vi "new_plot.vi"(10 "簇":T1, 11 "配置输入":T2 {"串口通信UI"."Format" items=["标准帧", "扩展帧"]; "串口通信UI"."Type" items=["数据帧", "远程帧"]; "串口通信UI"."ID" format="0x%x"; "串口通信UI"."Fliter" items=["接收所有类型"=1, "只接收标准帧"=2, "只接收扩展帧"=3]; "串口通信UI"."kBaudRate" items=["5k bps"=1, "10k bps"=2, "20k bps"=3, "40k bps"=4, "50k bps"=5, "80k bps"=6, "100k bps"=7, "125k bps"=8, "200k bps"=9, "250k bps"=10, "400k bps"=11, "500k bps"=12, "666k bps"=13, "800k bps"=14, "1000k bps"=15, "33.33k bps"=16, "66.66k bps"=17, "83.33k bps"=18]; "串口通信UI"."Mode" items=["正常工作", "仅侦听模式", "自测模式（环回）"]; "串口通信UI"."InitFlag" items=["使用界面设置参数"=1]; "串口通信UI"."AccMask" format="%08x"; "串口通信UI"."AccCode" format="%08x"; "串口通信UI"."Channel" items=["通道1", "通道2"]; "串口通信UI"."DevType" items=["USB-CAN"=3, "USB-CAN2"=4]; "安全报警UI"."操作 8" items=["产生报警信息（不发声），等待手动操作", "产生报警信息（发声），等待手动操作", "产生报警信息（不发声），自动刹车", "产生报警信息（发声），自动刹车", "产生报警信息（不发声），立即自动断电，开启泄放电阻", "产生报警信息（发声），立即自动断电，开启泄放电阻"]; "安全报警UI"."操作 7" items=["产生报警信息（不发声），等待手动操作", "产生报警信息（发声），等待手动操作", "产生报警信息（不发声），自动刹车", "产生报警信息（发声），自动刹车", "产生报警信息（不发声），立即自动断电，开启泄放电阻", "产生报警信息（发声），立即自动断电，开启泄放电阻"]; "安全报警UI"."操作 6" items=["产生报警信息（不发声），等待手动操作", "产生报警信息（发声），等待手动操作", "产生报警信息（不发声），自动刹车", "产生报警信息（发声），自动刹车", "产生报警信息（不发声），立即自动断电，开启泄放电阻", "产生报警信息（发声），立即自动断电，开启泄放电阻"]; "安全报警UI"."操作 5" items=["产生报警信息（不发声），等待手动操作", "产生报警信息（发声），等待手动操作", "产生报警信息（不发声），自动刹车", "产生报警信息（发声），自动刹车", "产生报警信息（不发声），立即自动断电，开启泄放电阻", "产生报警信息（发声），立即自动断电，开启泄放电阻"]; "安全报警UI"."操作 4" items=["产生报警信息（不发声），等待手动操作", "产生报警信息（发声），等待手动操作", "产生报警信息（不发声），自动刹车", "产生报警信息（发声），自动刹车", "产生报警信息（不发声），立即自动断电，开启泄放电阻", "产生报警信息（发声），立即自动断电，开启泄放电阻"]; "安全报警UI"."操作 3" items=["产生报警信息（不发声），等待手动操作", "产生报警信息（发声），等待手动操作", "产生报警信息（不发声），自动刹车", "产生报警信息（发声），自动刹车", "产生报警信息（不发声），立即自动断电，开启泄放电阻", "产生报警信息（发声），立即自动断电，开启泄放电阻"]; "安全报警UI"."操作 2" items=["产生报警信息（不发声），等待手动操作", "产生报警信息（发声），等待手动操作", "产生报警信息（不发声），自动刹车", "产生报警信息（发声），自动刹车", "产生报警信息（不发声），立即自动断电，开启泄放电阻", "产生报警信息（发声），立即自动断电，开启泄放电阻"]; "安全报警UI"."操作" items=["产生报警信息（不发声），等待手动操作", "产生报警信息（发声），等待手动操作", "产生报警信息（不发声），自动刹车", "产生报警信息（发声），自动刹车", "产生报警信息（不发声），立即自动断电，开启泄放电阻", "产生报警信息（发声），立即自动断电，开启泄放电阻"]}) -> (3 "配置输出":T2 {"串口通信UI"."Format" items=["标准帧", "扩展帧"]; "串口通信UI"."Type" items=["数据帧", "远程帧"]; "串口通信UI"."ID" format="0x%x"; "串口通信UI"."Fliter" items=["接收所有类型"=1, "只接收标准帧"=2, "只接收扩展帧"=3]; "串口通信UI"."kBaudRate" items=["5k bps"=1, "10k bps"=2, "20k bps"=3, "40k bps"=4, "50k bps"=5, "80k bps"=6, "100k bps"=7, "125k bps"=8, "200k bps"=9, "250k bps"=10, "400k bps"=11, "500k bps"=12, "666k bps"=13, "800k bps"=14, "1000k bps"=15, "33.33k bps"=16, "66.66k bps"=17, "83.33k bps"=18]; "串口通信UI"."Mode" items=["正常工作", "仅侦听模式", "自测模式（环回）"]; "串口通信UI"."InitFlag" items=["使用界面设置参数"=1]; "串口通信UI"."AccMask" format="%08x"; "串口通信UI"."AccCode" format="%08x"; "串口通信UI"."Channel" items=["通道1", "通道2"]; "串口通信UI"."DevType" items=["USB-CAN"=3, "USB-CAN2"=4]; "安全报警UI"."操作 8" items=["产生报警信息（不发声），等待手动操作", "产生报警信息（发声），等待手动操作", "产生报警信息（不发声），自动刹车", "产生报警信息（发声），自动刹车", "产生报警信息（不发声），立即自动断电，开启泄放电阻", "产生报警信息（发声），立即自动断电，开启泄放电阻"]; "安全报警UI"."操作 7" items=["产生报警信息（不发声），等待手动操作", "产生报警信息（发声），等待手动操作", "产生报警信息（不发声），自动刹车", "产生报警信息（发声），自动刹车", "产生报警信息（不发声），立即自动断电，开启泄放电阻", "产生报警信息（发声），立即自动断电，开启泄放电阻"]; "安全报警UI"."操作 6" items=["产生报警信息（不发声），等待手动操作", "产生报警信息（发声），等待手动操作", "产生报警信息（不发声），自动刹车", "产生报警信息（发声），自动刹车", "产生报警信息（不发声），立即自动断电，开启泄放电阻", "产生报警信息（发声），立即自动断电，开启泄放电阻"]; "安全报警UI"."操作 5" items=["产生报警信息（不发声），等待手动操作", "产生报警信息（发声），等待手动操作", "产生报警信息（不发声），自动刹车", "产生报警信息（发声），自动刹车", "产生报警信息（不发声），立即自动断电，开启泄放电阻", "产生报警信息（发声），立即自动断电，开启泄放电阻"]; "安全报警UI"."操作 4" items=["产生报警信息（不发声），等待手动操作", "产生报警信息（发声），等待手动操作", "产生报警信息（不发声），自动刹车", "产生报警信息（发声），自动刹车", "产生报警信息（不发声），立即自动断电，开启泄放电阻", "产生报警信息（发声），立即自动断电，开启泄放电阻"]; "安全报警UI"."操作 3" items=["产生报警信息（不发声），等待手动操作", "产生报警信息（发声），等待手动操作", "产生报警信息（不发声），自动刹车", "产生报警信息（发声），自动刹车", "产生报警信息（不发声），立即自动断电，开启泄放电阻", "产生报警信息（发声），立即自动断电，开启泄放电阻"]; "安全报警UI"."操作 2" items=["产生报警信息（不发声），等待手动操作", "产生报警信息（发声），等待手动操作", "产生报警信息（不发声），自动刹车", "产生报警信息（发声），自动刹车", "产生报警信息（不发声），立即自动断电，开启泄放电阻", "产生报警信息（发声），立即自动断电，开启泄放电阻"]; "安全报警UI"."操作" items=["产生报警信息（不发声），等待手动操作", "产生报警信息（发声），等待手动操作", "产生报警信息（不发声），自动刹车", "产生报警信息（发声），自动刹车", "产生报警信息（不发声），立即自动断电，开启泄放电阻", "产生报警信息（发声），立即自动断电，开启泄放电阻"]})   [LabVIEW 2018, in "UI.lvlib"]
uses:
  UI.lvlib
  Settings/Settings.ctl
  Acquisition/Hardware Configuration.ctl
  Acquisition/Signal Type.ctl
  Logging/Logging Configuration.ctl
  Logging/Logging.lvlib
  Acquisition/Acquisition.lvlib
  Settings/Settings.lvlib
panel:
  # "参数配置文件"
  # "输入数据文件"
  # "加载电机"
  # "负载电机"
  # "注：每次运行实验时销毁现有所有图像"
  # "参数配置文件"
  # "输入数据文件"
  # "加载电机"
  # "负载电机"
  # "注：每次运行实验时销毁现有所有图像"
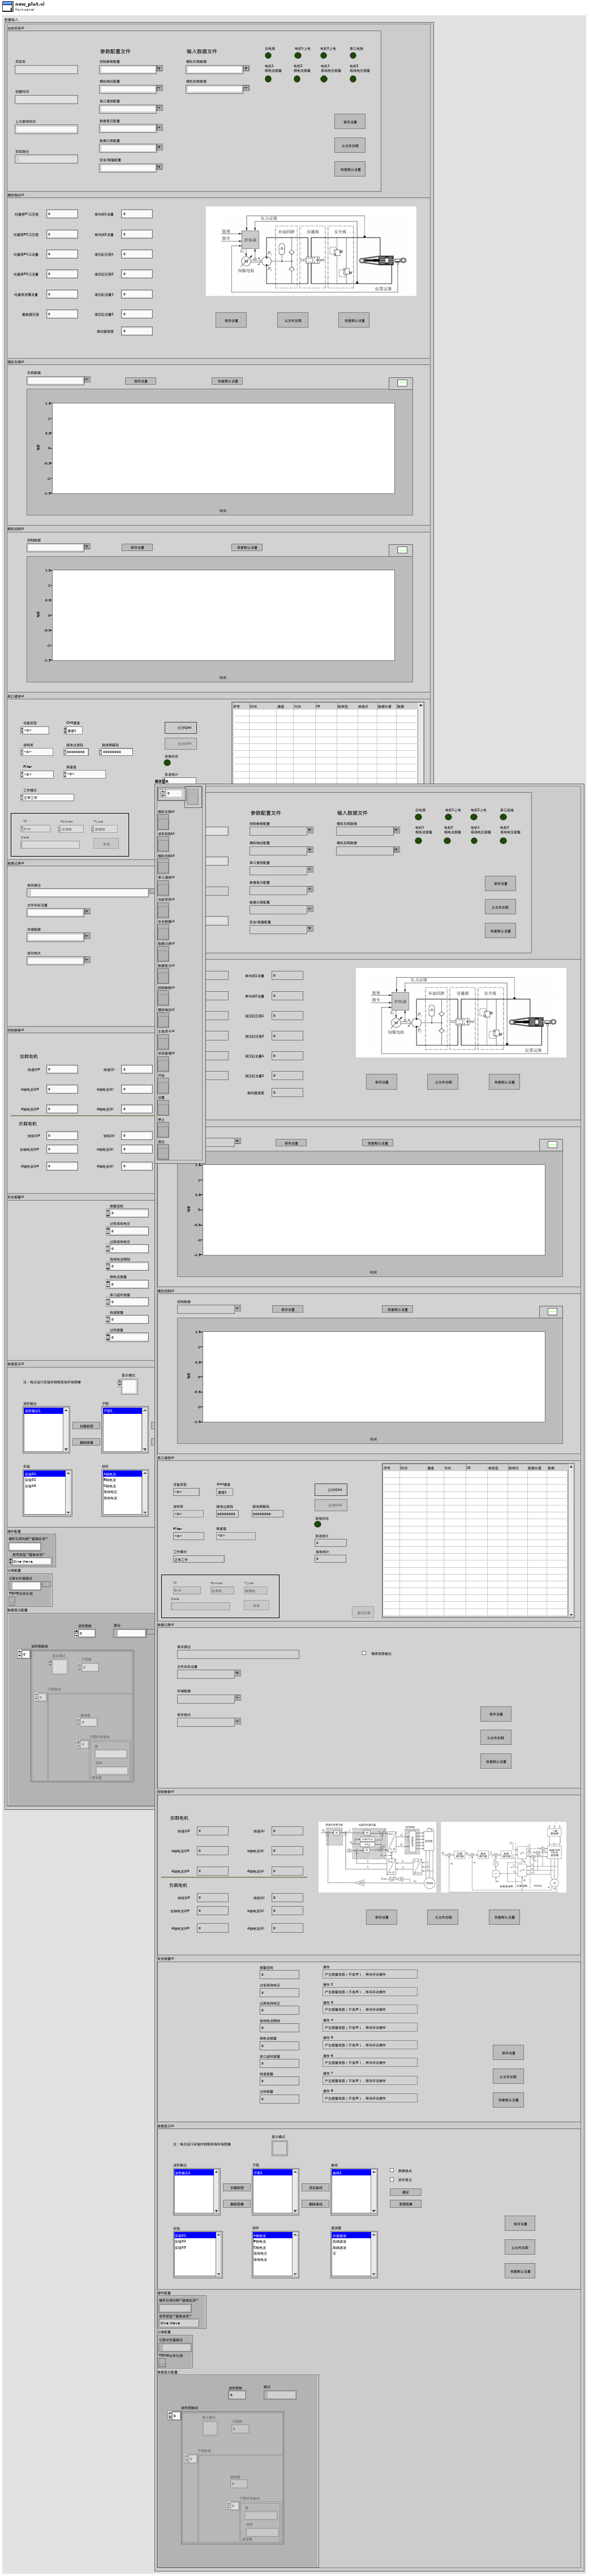
[diagram p1: front panel]
types:
  T1 = typedef "引用簇.ctl" = cluster{"数组":refnum<vi>[], "模拟负载UI":refnum<vi>, "波形控制UI":refnum<vi>, "模拟控制UI":refnum<vi>, "串口通信UI":refnum<vi>, "当前项目UI":refnum<vi>, "安全报警UI":refnum<vi>, "数据记录UI":refnum<vi>, "数据显示UI":refnum<vi>, "控制参数UI":refnum<vi>, "模拟响应UI":refnum<vi>, "主选项卡UI":refnum<vi>, "项目管理UI":refnum<vi>, "开始":refnum<vi>, "设置":refnum<vi>, "停止":refnum<vi>, "退出":refnum<vi>}
  T2 = typedef "Settings.lvlib/Settings.ctl" = cluster{"当前项目UI":T3, "模拟响应UI":T4, "模拟负载UI":T5, "模拟控制UI":T6, "串口通信UI":T7, "数据记录UI":T13, "控制参数UI":T14, "安全报警UI":T15, "数据显示UI":T16, "硬件配置":T17, "记录配置":T19, "数据显示配置":T20}
  T3 = typedef "控件 5.ctl" = cluster{"控制参数配置":string, "模拟响应配置":string, "串口通信配置":string, "数据显示配置":string, "数据记录配置":string, "安全/报警配置":string, "模拟负载数据":string, "模拟加载数据":string, "总电源":bool, "电机1上电":bool, "电机2上电":bool, "串口连接":bool, "电机1\n相电流报警":bool, "电机2\n相电流报警":bool, "电机1\n母线电压报警":bool, "电机2\n母线电压报警":bool, "保存设置":bool, "从文件加载":bool, "恢复默认设置":bool, "路径":path, "项目路径":path, "项目名":string, "创建时间":string, "上次使用时间":string}
  T4 = typedef "模拟响应UI.ctl" = cluster{"柱塞泵P!口压强":dbl, "柱塞泵P2口压强":dbl, "柱塞泵P1口流量":dbl, "柱塞泵P2口流量":dbl, "柱塞泵泄露流量":dbl, "蓄能器压强":dbl, "单向阀1流量":dbl, "单向阀2流量":dbl, "液压缸压强1":dbl, "液压缸压强2":dbl, "液压缸流量1":dbl, "液压缸流量2":dbl, "做动器速度":dbl, "保存设置":bool, "从文件加载":bool, "恢复默认设置":bool, "路径":path}
  T5 = typedef "控件 9.ctl" = cluster{"负载数据":string, "负载数据 2":waveform(dbl)[], "保存设置":bool, "恢复默认设置":bool}
  T6 = typedef "控件 7.ctl" = cluster{"控制数据":string, "负载数据 2":waveform(dbl)[], "保存设置":bool, "恢复默认设置":bool}
  T7 = typedef "控件 6.ctl" = cluster{"DevType":T8, "Channel":T9, "AccCode":u32, "AccMask":u32, "InitFlag":T10, "Mode":T11, "kBaudRate":u8, "Fliter":T12, "Open":bool, "Close":bool, "连接状态":bool, "SendCnt":u32, "RecvCnt":u32, "Send":bool, "ID":u32, "Data":string, "Type":u8, "Format":u8, "Clear":bool, "list":i32, "路径":path}
  T8 = typedef "ControlCAN.lvlib/DevType.ctl" = u32
  T9 = typedef "ControlCAN.lvlib/CAN Channel.ctl" = u32
  T10 = typedef "ControlCAN.lvlib/InitFlag.ctl" = u32
  T11 = typedef "ControlCAN.lvlib/Mode.ctl" = u8
  T12 = typedef "ControlCAN.lvlib/Fliter.ctl" = u8
  T13 = typedef "控件 3.ctl" = cluster{"保存路径":path, "文件命名设置":string, "存储数据":string, "保存格式":string, "复选框":bool, "保存设置":bool, "从文件加载":bool, "恢复默认设置":bool, "路径":path}
  T14 = typedef "控件 1.ctl" = cluster{"d轴电流环P":dbl, "转速环P":dbl, "q轴电流环P":dbl, "d轴电流环P":dbl, "转矩环P":dbl, "去轴电流环P":dbl, "转速环I":dbl, "q轴电流环I":dbl, "d轴电流环I":dbl, "转矩环I":dbl, "q轴电流环I":dbl, "d轴电流环I":dbl, "保存设置":bool, "从文件加载":bool, "恢复默认设置":bool, "路径":path}
  T15 = typedef "控件 4.ctl" = cluster{"报警扭矩":dbl, "过低母线电压":dbl, "过高母线电压":dbl, "母线电流限制":dbl, "相电流报警":dbl, "串口超时报警":dbl, "转速报警":dbl, "过热报警":dbl, "操作":u16, "操作 2":u16, "操作 3":u16, "操作 4":u16, "操作 5":u16, "操作 6":u16, "操作 7":u16, "操作 8":u16, "保存设置":bool, "从文件加载":bool, "恢复默认设置":bool, "路径":path}
  T16 = typedef "控件 2.ctl" = cluster{"保存设置":bool, "从文件加载":bool, "恢复默认设置":bool, "实验":i32, "波形输出":i32, "组件":i32, "曲线":i32, "滤波器":i32, "删除曲线":bool, "清理图像":bool, "添加曲线":bool, "数据选点":bool, "确定按钮":bool, "实时显示":bool, "子图":i32, "显示模式":u16, "路径":path, "删除图像":bool, "创建新图":bool}
  T17 = typedef "Acquisition.lvlib/Hardware Configuration.ctl" = cluster{"硬件引用句柄<替换此项>":string, "信号类型<替换该项>":T18}
  T18 = typedef "Acquisition.lvlib/Signal Type.ctl" = enum16{"Sine Wave", "Square with Noise"}
  T19 = typedef "Logging.lvlib/Logging Configuration.ctl" = cluster{"记录文件基路径":path, "TDMS文件引用":refnum<k34>}
  T20 = typedef "波形图簇.ctl" = cluster{"波形图数":u32, "波形图数组":T21[], "路径":path}
  T21 = typedef "波形图.ctl" = cluster{"显示模式":u16, "子图数":u32, "子图数组":T22[]}
  T22 = typedef "子图.ctl" = cluster{"子图所有曲线":T23[], "曲线数":u32}
  T23 = typedef "曲线簇.ctl" = cluster{"源":string, "组件":string, "滤波器":string}
  T24 = enum8{"Enabled", "Disabled", "Disabled and Grayed Out"}
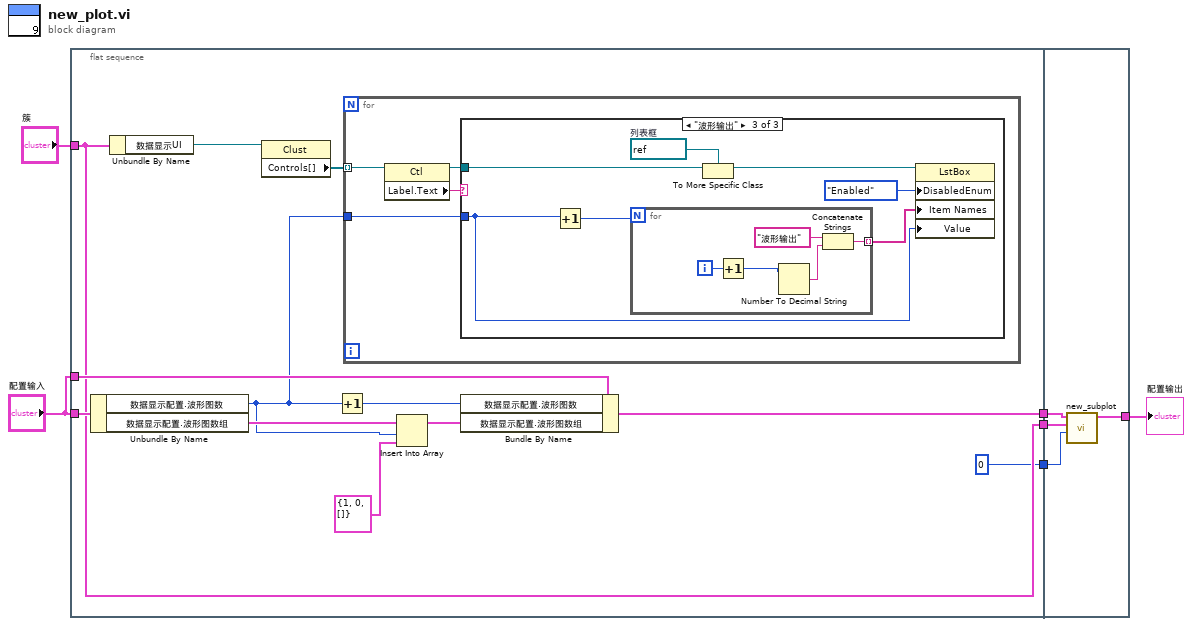
[diagram p0: block diagram]
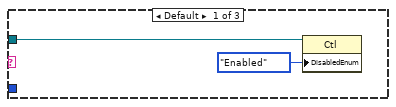
[diagram p2: hidden frame]
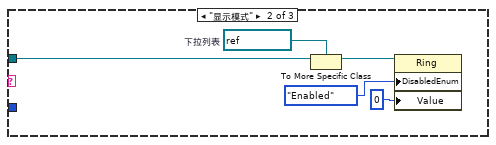
[diagram p3: hidden frame]
diagram:
  n1 = flat-sequence {
    tunnel: "簇" -> [w12]
    tunnel: "配置输入" -> [w16]
    tunnel: "配置输入" -> [w14]
    tunnel: [w13] -> w4
    tunnel: [w12] -> w2
    tunnel: [0] -> w1
    tunnel: [w45] -> w3
    tunnel: w4 -> [w44]
    tunnel: w2 -> [w43]
    tunnel: w1 -> [w42]
    frame #0 {
      n2 = Unbundle By Name(w16) -> ("数据显示配置.波形图数"=w8:u32, "数据显示配置.波形图数组"=w11:T21[])
      n3 = Unbundle By Name(w12) -> ("数据显示UI"=w17:refnum<vi>)
      n4 = property class="Clust"(reference=w17) -> ("Controls[]"=w18:refnum<vi>[])  [unwired: 1 in, 2 out]
      n5 = Increment(x=w8) -> (x+1=w15:u32)
      n6 = for {
        tunnel: w18 -> [w22] mode=indexing
        tunnel: w8 -> [w19]
        n7 = property class="Ctl"(reference=w22) -> (reference out=w20:refnum<vi>, "Label.Text"=w21:string)  [unwired: 1 in, 1 out]
        n8 = case shown="\"波形输出\"" w21 {
          tunnel: w20 -> [w24 w27 w35]
          tunnel: w19 -> [_ _ w31]
          frame Default {
            n9 = property class="Ctl"(reference=w24, "DisabledEnum"=T24."Enabled" ("禁用")) -> ()  [unwired: 1 in, 2 out]
          }
          frame "显示模式" {
            w28 = refnum<vi> refnum  # 下拉列表
            n10 = To More Specific Class(target class=w28, reference=w27) -> (specific class reference=w26:refnum<vi>)  [unwired: 1 in, 1 out]
            n11 = property class="Ring"(reference=w26, "DisabledEnum"=T24."Enabled" ("禁用"), "Value"=0) -> ()  [unwired: 1 in, 2 out]
          }
          frame "波形输出" {
            w34 = refnum<vi> refnum  # 列表框
            n12 = Increment(x=w31) -> (x+1=w30:u32)
            n13 = for {
              N: w30 -> [_]
              tunnel: [w39] -> w32 mode=indexing
              i -> [w41]
              n14 = Increment(x=w41) -> (x+1=w37:i32)
              n15 = Number To Decimal String(number=w37) -> (decimal integer string=w38:string)  [unwired: 1 in]
              n16 = Concatenate Strings("波形输出", w38) -> (w39:string)
            }
            n17 = To More Specific Class(target class=w34, reference=w35) -> (specific class reference=w33:refnum<vi>)  [unwired: 1 in, 1 out]
            n18 = property class="LstBox"(reference=w33, "DisabledEnum"=T24."Enabled" ("禁用"), "Item Names"=w32, "Value"=w31) -> ()  [unwired: 1 in, 2 out]
          }
        }
      }
      n19 = Insert Into Array(array=w11, index=w8, new element=T21 {"显示模式"=1, "子图数"=0, "子图数组"=[]} ("波形图")) -> (w9:T21[])
      n20 = Bundle By Name(cluster=w14, "数据显示配置.波形图数"=w15, "数据显示配置.波形图数组"=w9) -> (w13:T2)
    }
    frame #1 {
      n21 = call "new_subplot.vi"("显示模式"=w42, "簇"=w43, "配置输入"=w44) -> ("配置输出"=w45:T2)  [unwired: 8 in]
    }
  }
  "配置输出" <- w3
